vi "get channels.vi"(11 "Profibus Module configuration in":refnum<class "Profibus Module configuration.lvclass">) -> (2 "channels":refnum<class "TBM channel.lvclass">[](array[class]), 3 "Profibus Module configuration out":refnum<class "Profibus Module configuration.lvclass">)   [LabVIEW 2013, in "Profibus Module configuration.lvclass"]
uses:
  Profibus Module configuration.lvclass
  <vilib>/NI/Tag Bus Module Framework/channel/TBM channel.lvclass
  Profibus Module configuration.lvclass/Profibus Module configuration.ctl
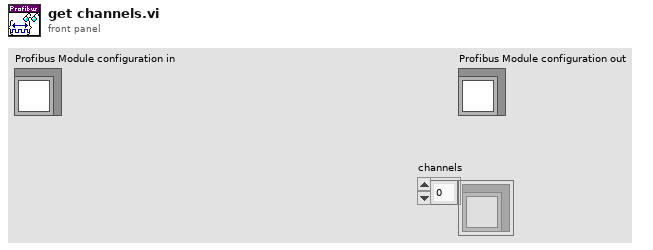
[diagram p1: front panel]
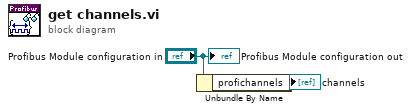
[diagram p0: block diagram]
diagram:
  n1 = Unbundle By Name("Profibus Module configuration in") -> ("profichannels"=→"channels":refnum<class "Profibus channel.lvclass">[])
  "Profibus Module configuration out" <- "Profibus Module configuration in"
